vi "LI-U8 check if equal.vi"(3 "Large number - U8 B":T1, 5 "Large number - U8 A":T1) -> (2 "Equal?":bool)   [LabVIEW 2009]
doc: "Subtracts two large numbers (U8 array format). Then checks if result = 0. If so, output 'equal?\" = T."
uses:
  User Access Type defs/Large number - U8 array.ctl
panel:
  # "index 0 = LSD"
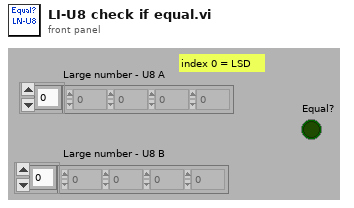
[diagram p1: front panel]
types:
  T1 = typedef "Large number - U8 array.ctl" = u8[]
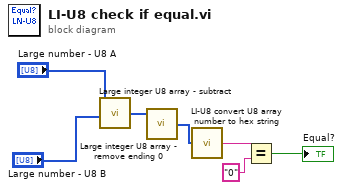
[diagram p0: block diagram]
diagram:
  n1 = call "Large integer U8 array - subtract.vi"("Large number - U8 B"="Large number - U8 B", "Large number - U8 A"="Large number - U8 A") -> ("A-B"=w5:T1)  [unwired: 3 out]
  n2 = call "Large integer U8 array - remove ending 0.vi"("Large number - U8"=w5) -> ("MSD zeros removed"=w4:T1)  [unwired: 4 out]
  n3 = call "LI-U8 convert U8 array number to hex string.vi"("Large number -U8"=w4) -> ("hex string (MSD 1st)"=w3:string)  [unwired: 4 out]
  n4 = Equal?(x=w3, y="0") -> (x = y?=→"Equal?":bool)
